vi "Nelson_Whale_Coords.vi"(3 "error in (no error)":errorcluster, 4 "Color Based Tracking?":bool, 5 "Image":T1(plugin-control)) -> (0 "error out":errorcluster, 1 "Position":cluster{"Y":dbl, "X":dbl}, 2 "Image Out":T1(plugin-control))   [LabVIEW 2014]
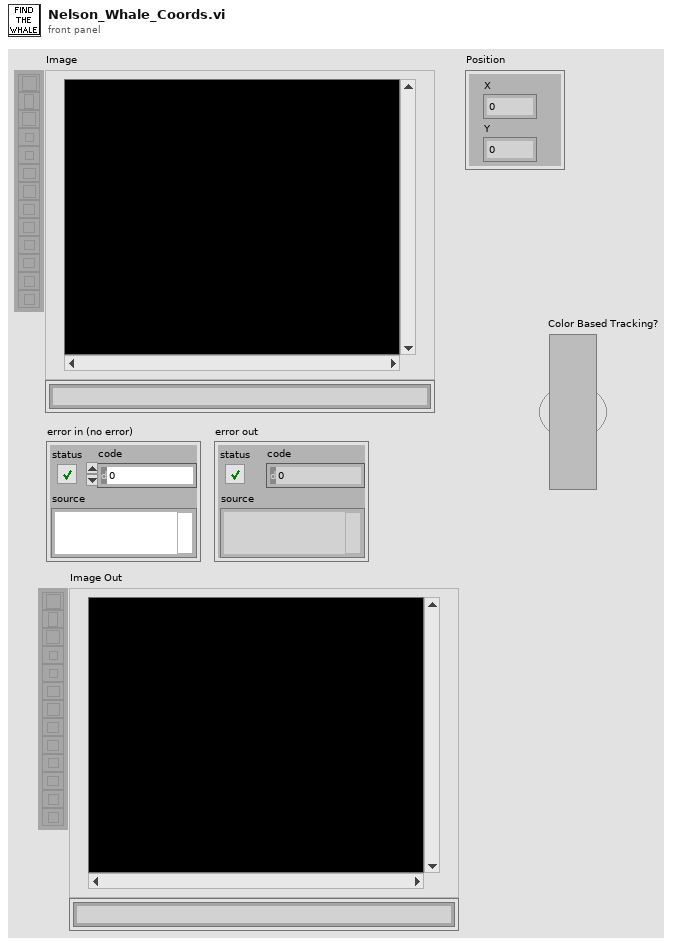
[diagram p1: front panel]
types:
  T1 = typedef "IMAQ Image.ctl" = refnum<image>
  T2 = cluster{"Position":cluster{"x":sgl, "y":sgl}, "Angle":sgl, "Scale":sgl, "Score":sgl, "Bounding Box":cluster{"x":sgl, "y":sgl}[]}[]
  T3 = cluster{"Position":cluster{"x":sgl, "y":sgl}, "Angle":sgl, "Scale":sgl, "Score":sgl, "Bounding Box":cluster{"x":sgl, "y":sgl}[]}
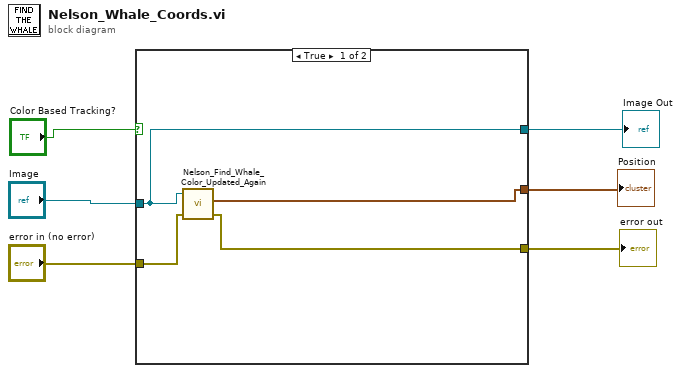
[diagram p0: block diagram]
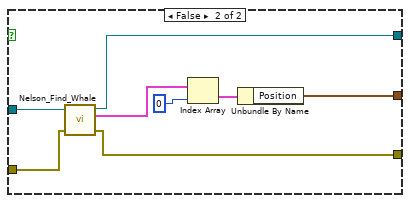
[diagram p2: hidden frame]
diagram:
  n1 = case shown="True" "Color Based Tracking?" {
    tunnel: [w9 w18] -> w6
    tunnel: [w8 w15] -> w5
    tunnel: "error in (no error)" -> [w10 w14]
    tunnel: "Image" -> [w7 w13]
    tunnel: [w7 w12] -> w2
    frame True {
      n2 = call "Nelson_Find_Whale_Color_Updated_Again.vi"("error in"=w10, "Image In"=w7) -> ("error out"=w9:errorcluster, "Calibrated Centroid (Centroid 1)"=w8:cluster{"X Centroid":sgl, "Y Centroid":sgl})  [unwired: 1 in, 1 out]
    }
    frame False {
      n3 = call "Nelson_Find_Whale.vi"("error in"=w14, "Image In"=w13) -> ("error out"=w18:errorcluster, "Matches (Color Location 1)"=w11:T2, "Image Out"=w12:T1)  [unwired: 1 in]
      n4 = Index Array(array=w11, index=0) -> (element=w16:T3)
      n5 = Unbundle By Name(w16) -> ("Position"=w15:cluster{"x":sgl, "y":sgl})
    }
  }
  "error out" <- w6
  "Position" <- w5
  "Image Out" <- w2
